vi "MIPI RFFE Write Waveform.vi"(0 "Data":T1 {"Register" format="%.0x"; "Slave Address" max=15 format="%.0x"}, 5 "Configuratation":T2={"Samples to Allocate"=10000, "Oversample Factor"=1, "Clock Channel"=enum."0", "Data Channel"=enum."1"} {"Oversample Factor" min=1 max=254; "Samples to Allocate" min=1}, 11 "error in (no error)":errorcluster) -> (6 "Waveform Graph":digitalwaveform(graph), 15 "error out":errorcluster)   [LabVIEW 2013]
uses:
  Ctrls/Configuration.ctl
  Ctrls/ClockDataChannels.ctl
  Ctrls/RegReadWrite.ctl
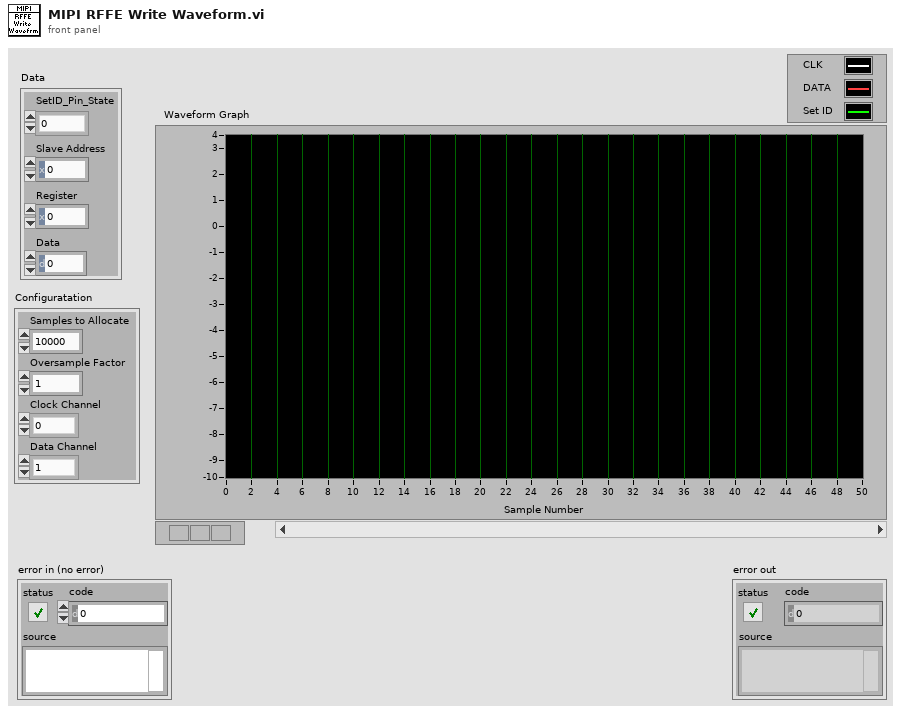
[diagram p1: front panel]
types:
  T1 = typedef "RegReadWrite.ctl" = cluster{"Slave Address":u8, "Register":u8, "Data":u8, "SetID_Pin_State":enum16{"0", "1", "Z"}}
  T2 = typedef "Configuration.ctl" = cluster{"Samples to Allocate":i32, "Oversample Factor":u8, "Clock Channel":T3, "Data Channel":T3}
  T3 = typedef "ClockDataChannels.ctl" = enum16{"0", "1"}
  T4 = typedef "RFFE_Data.ctl" = cluster{"Clock Channel":T3, "Data Channel":T3, "Oversample Factor":u8, "Zero Array":u8[], "One Array":u8[], "Z Array ":u8[], "H Array":u8[], "L Array":u8[], "X Array":u8[], "Toggle (high to low)":u8[]}
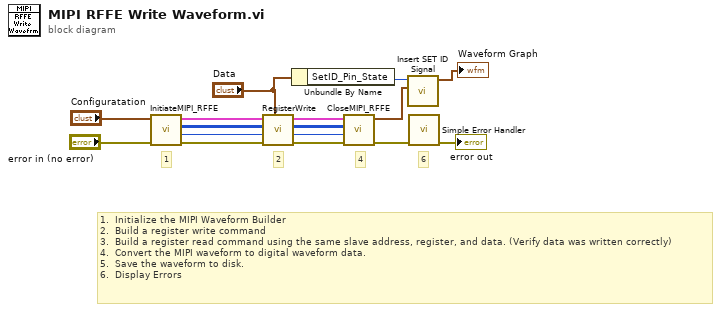
[diagram p0: block diagram]
diagram:
  # "6"
  # "1.  Initialize the MIPI Waveform Builder\n2.  Build a register write command\n3.  Build a register read command using the same slave address, register, and data. (Verify data was written correctly)\n4.  Convert the MIPI waveform to digital waveform data.\n5.  Save the waveform to disk.\n6.  Display Errors"
  # "4"
  # "2"
  # "1"
  n1 = call "InitiateMIPI_RFFE.vi"("error in (no error)"="error in (no error)", "Configuratation In"="Configuratation") -> ("error out"=w16:errorcluster, "Number of Samples Out"=w14:i32, "Data Array"=w13:u8[][], "RFFE_Data"=w15:T4)  [unwired: 6 in]
  n2 = call "RegisterWrite.vi"("Write Data"="Data", "error in (no error)"=w16, "Number of Samples In"=w14, "Data Array"=w13, "RFFE_Data"=w15) -> ("error out"=w8:errorcluster, "Number of Samples Out"=w9:i32, "Data Array Out"=w10:u8[][], "Configuratation Out"=w11:T4)  [unwired: 3 in]
  n3 = Unbundle By Name("Data") -> ("SetID_Pin_State"=w1:enum16{"0", "1", "Z"})
  n4 = call "CloseMIPI_RFFE.vi"("error in (no error)"=w8, "Number of Samples"=w9, "Data Array"=w10, "RFFE_Data"=w11) -> ("error out"=w7:errorcluster, "Digital Waveform"=w3:digitalwaveform)  [unwired: 6 in]
  n5 = call "Insert SET ID Signal.vi"("Digital Waveform Graph"=w3, "SetID_Pin_State"=w1) -> ("Digital Waveform Graph 2"=→"Waveform Graph":digitalwaveform)  [unwired: 9 in]
  n6 = call <vilib>:"Simple Error Handler.vi"("error in (no error)"=w7) -> ("error out"=→"error out":errorcluster)  [unwired: 4 in, 4 out]
